vi "Measurement Logic.vi"() -> ()   [LabVIEW 2024, in "Broadband Generation.lvlib"]
uses:
  Broadband Generation.lvlib
  Measurement Results.ctl
  <vilib>/addons/_NISVFA/_Generation/Signal Generation/SV Signal/sv_System Timing Model.ctl
  <vilib>/addons/_NISVFA/_Generation/Signal Generation/SV Signal/SV Signal.lvclass
  <vilib>/addons/_NISVFA/_Generation/Signal Generation/SV Sinusoid/SV Sinusoid.lvclass
  <resource>/objmgr/daqmx.rc
  <vilib>/DAQmx/configure/timing.llb/DAQmx Timing (Sample Clock).vi
  <vilib>/addons/_NISVFA/_Generation/Signal Generation/SV Noise/Configure White Noise.vi
  <vilib>/addons/_NISVFA/_Generation/Signal Generation/SV Noise/SV Noise.lvclass
  <vilib>/DAQmx/create/channels.llb/DAQmx Create Channel (AO-Voltage-Basic).vi
  <vilib>/DAQmx/write.llb/DAQmx Write (Analog 1D Wfm NChan NSamp).vi
  <vilib>/addons/_NISVFA/_Generation/Signal Generation/SV Noise/Configure Pink Noise.vi
  <vilib>/addons/_NISVFA/_Generation/Signal Generation/SV Noise/Configure Periodic Random Noise.vi
  <vilib>/addons/_NISVFA/_Generation/Signal Generation/SV MLS/Configure Maximum Length Sequence.vi
  <vilib>/addons/_NISVFA/_Generation/Signal Generation/SV MLS/SV MLS.lvclass
  <vilib>/Plug-In SDKs/Measurements/Measure Call Context/Measure Call Context.lvclass
  Measurement Configuration.ctl
panel:
  out "measurement results":T1
  in  "measurement configuration":T2={"sample rate"=51200.0, "physical channels"=["Dev1/ao0"], "ranges"=[3.16], "terminal cfgs"=[-1], "type"=[0], "levels"=[0.5]} {"type" items=["White Noise", "Pink Noise", "Periodic Random Noise", "Maximum Length Sequence"]}
  out "measure call context out":refnum<class "Measure Call Context.lvclass">
  in  "measure call context in":refnum<class "Measure Call Context.lvclass">
  out "error out":errorcluster
  in  "error in":errorcluster
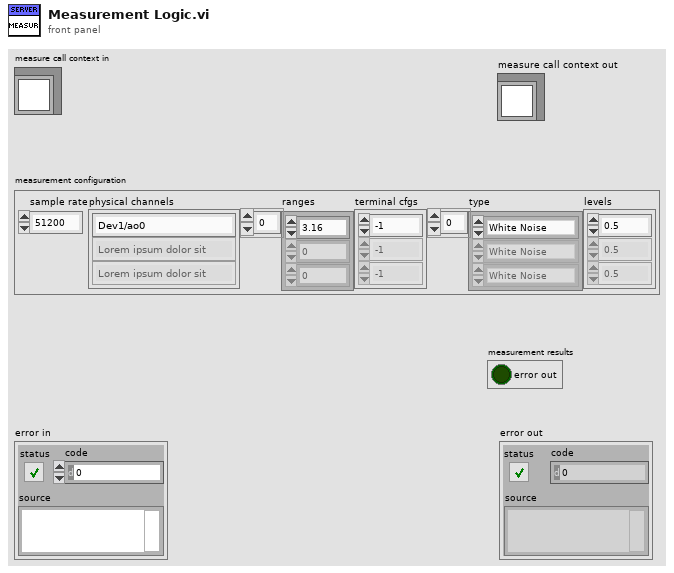
[diagram p1: front panel]
types:
  T1 = typedef "Broadband Generation.lvlib/Measurement Results.ctl" = cluster{"error out":bool}
  T2 = typedef "Broadband Generation.lvlib/Measurement Configuration.ctl" = cluster{"sample rate":dbl, "physical channels":string[], "ranges":dbl[], "terminal cfgs":i32[], "type":i32[], "levels":dbl[]}
  T3 = cluster{"profile":enum16{"Linear", "Half cosine"}, "durations [s]":cluster{"ramp-up":dbl, "transition":dbl, "ramp-down":dbl}}
  T4 = typedef "SV Signal.lvclass/sv_System Timing Model.ctl" = i64
  T5 = typedef "Event Messenger-bool.lvlib/))Channel.ctl" = refnum<queue>
  T6 = typedef "Tag-bool.lvlib/))Channel.ctl" = refnum<queue>
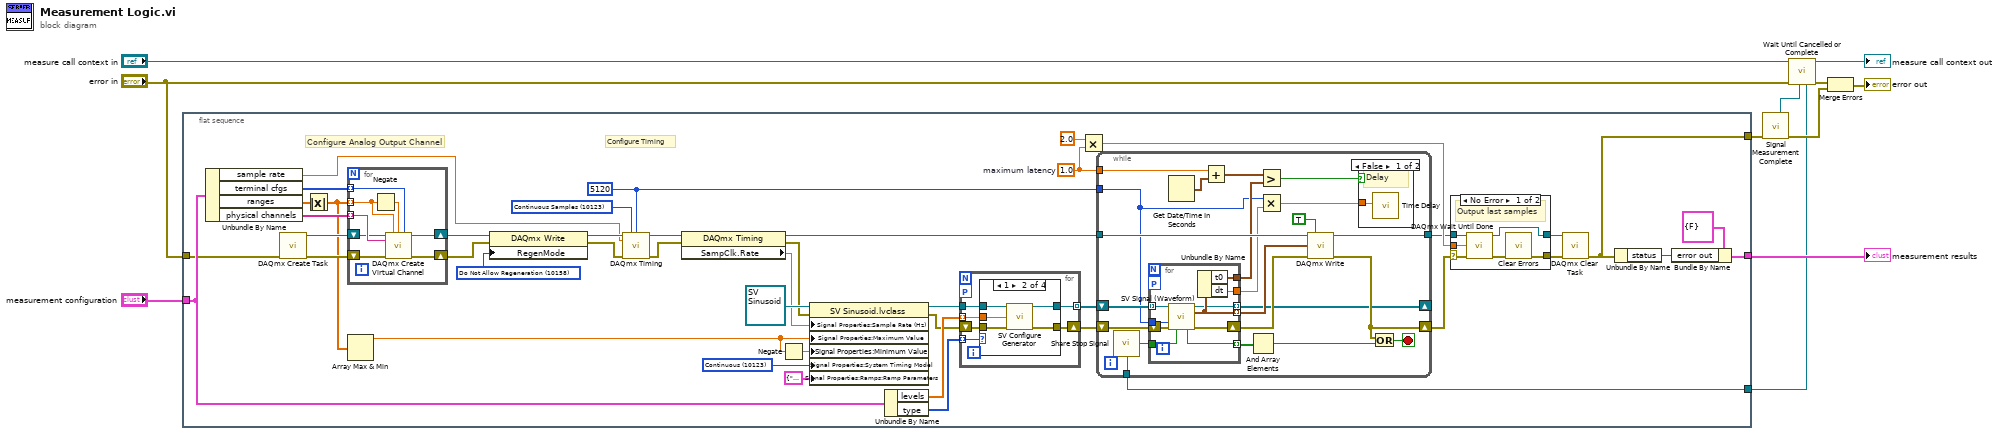
[diagram p0: block diagram]
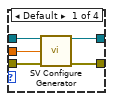
[diagram p4: hidden frame]
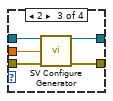
[diagram p5: hidden frame]
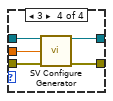
[diagram p6: hidden frame]
diagram:
  n1 = flat-sequence {
    tunnel: "measurement configuration" -> [w53]
    tunnel: [w55] -> w5
    tunnel: "error in" -> [w23]
    tunnel: [w20] -> w3
    tunnel: w4 -> [w24]
    frame #0 {
      w35 = 10158 items=["Allow Regeneration"=10097, "Do Not Allow Regeneration"=10158] ("RegenMode")
      w18 = 5120 ("samples per channel")
      w43 = 10123 items=["Finite Samples"=10178, "Continuous Samples"=10123, "Hardware Timed Single Point"=12522] ("sample mode")
      w28 = 1.0  # maximum latency
      w54 = T4 10123 items=["Finite"=10178, "-"=-1, "Continuous"=10123, "-"=-2, "Settled"=110123, "Averaged"=210123, "Discrete Sweep"=310123, "Continuous Sweep"=410123] ("System Timing Model")
      # "Configure Timing"
      # "Configure Analog Output Channel"
      n2 = Unbundle By Name(w53) -> ("sample rate"=w22:dbl, "terminal cfgs"=w36:i32[], "ranges"=w15:dbl[], "physical channels"=w37:string[])
      n3 = call <vilib>:"DAQmx Create Task.vi"("error in"=w23) -> ("task out"=w34:refnum<k21>, "error out"=w33:errorcluster)  [unwired: 13 in]
      n4 = Absolute Value(x=w15) -> (abs(x)=w14:dbl[])
      n5 = for {
        tunnel: w37 -> [w101] mode=indexing
        tunnel: w14 -> [w100] mode=indexing
        tunnel: w36 -> [w99] mode=indexing
        shift-right: [w103] -> w41
        shift-left: w34 -> [w98]
        shift-right: [w102] -> w39
        shift-left: w33 -> [w97]
        n6 = Negate(x=w100) -> (-x=w104:dbl)
        n7 = call-poly <vilib>:"DAQmx Create Virtual Channel.vi"("task in"=w98, "maximum value"=w100, "minimum value"=w104, "output terminal configuration"=w99, "physical channels"=w101, "error in"=w97) -> ("task out"=w103:refnum<k21>, "error out"=w102:errorcluster)  [unwired: 8 in]
      }
      n8 = Array Max & Min(array=w14) -> (max value=w12:dbl)  [unwired: 3 out]
      n9 = property class="DAQmx Write"(reference=w41, error in=w39, "RegenMode"=w35) -> (reference out=w40:refnum<k21>, error out=w38:errorcluster)
      n10 = call-poly <vilib>:"DAQmx Timing.vi"("task/channels in"=w40, "sample mode"=w43, "samples per channel"=w18, "rate"=w22, "error in"=w38) -> ("task out"=w44:refnum<k21>, "error out"=w42:errorcluster)  [unwired: 9 in]
      n11 = property class="DAQmx Timing"(reference=w44, error in=w42) -> (reference out=w27:refnum<k21>, error out=w31:errorcluster, "SampClk.Rate"=w32:dbl)
      n12 = Negate(x=w12) -> (-x=w13:dbl)
      n13 = property class="SV Sinusoid.lvclass"(reference=refnum<class "SV Sinusoid.lvclass"> refnum ("signal configuration"), error in=w31, "Signal Properties:Sample Rate (Hz)"=w32, "Signal Properties:Maximum Value"=w12, "Signal Properties:Minimum Value"=w13, "Signal Properties:System Timing Model"=w54, "Signal Properties:Ramps:Ramp Parameters"=T3 {"profile"=enum."Half cosine", "durations [s]"={"ramp-up"=0.01, "transition"=0.0, "ramp-down"=0.01}} ("Ramp Parameters:All Elements")) -> (reference out=w51:refnum<class "SV Sinusoid.lvclass">, error out=w48:errorcluster)
      n14 = Unbundle By Name(w53) -> ("levels"=w50:dbl[], "type"=w49:i32[])
      n15 = for {
        tunnel: w51 -> [w110]
        tunnel: w50 -> [w105] mode=indexing
        tunnel: w49 -> [w106] mode=indexing
        tunnel: [w109] -> w47 mode=indexing
        workers-P: _ -> [_]
        shift-right: [w108] -> w46
        shift-left: w48 -> [w107]
        n16 = case shown="1" w106 {
          tunnel: w110 -> [w115 w120 w125 w130]
          tunnel: [w114 w119 w124 w129] -> w109
          tunnel: [w113 w118 w123 w128] -> w108
          tunnel: w107 -> [w112 w117 w122 w127]
          tunnel: w105 -> [w111 w116 w121 w126]
          frame Default {
            n17 = call-poly <vilib>:"SV Configure Generator.vi"("template configuration"=w115, "level"=w111, "error in (no error)"=w112) -> ("signal configuration"=w114:refnum<class "SV Noise.lvclass">, "error out"=w113:errorcluster)  [unwired: 11 in]
          }
          frame 1 {
            n18 = call-poly <vilib>:"SV Configure Generator.vi"("template configuration"=w120, "level"=w116, "error in"=w117) -> ("signal configuration"=w119:refnum<class "SV Noise.lvclass">, "error out"=w118:errorcluster)  [unwired: 11 in]
          }
          frame 2 {
            n19 = call-poly <vilib>:"SV Configure Generator.vi"("template configuration"=w125, "level"=w121, "error in (no error)"=w122) -> ("signal configuration"=w124:refnum<class "SV Noise.lvclass">, "error out"=w123:errorcluster)  [unwired: 11 in]
          }
          frame 3 {
            n20 = call-poly <vilib>:"SV Configure Generator.vi"("template configuration"=w130, "amplitude"=w126, "error in (no error)"=w127) -> ("signal configuration"=w129:refnum<class "SV MLS.lvclass">, "error out"=w128:errorcluster)  [unwired: 11 in]
          }
        }
      }
      n21 = Multiply(x=2.0 ("value"), y=w28) -> (x*y=w29:dbl)
      n22 = while {
        tunnel: w28 -> [w59]
        tunnel: w27 -> [w73]
        shift-right: [w65] -> w25
        shift-left: w46 -> [w76]
        tunnel: [w70] -> w26
        tunnel: w24 -> [w69]
        shift-right: [w63] -> _
        shift-left: w47 -> [w77]
        tunnel: w18 -> [w56]
        stop <- w66 stop-if-true
        n23 = call <vilib>:"Share Stop Signal.vi"("channel"=w69) -> ("stop"=w68:bool)  [unwired: 1 in]
        n24 = for {
          tunnel: [w86] -> w74 mode=indexing
          workers-P: _ -> [_]
          tunnel: w77 -> [w88] mode=indexing
          tunnel: [w85] -> w57
          shift-right: [w84] -> w71
          shift-left: w76 -> [w87]
          tunnel: w68 -> [w83]
          tunnel: [w82] -> w67 mode=indexing
          tunnel: [w81] -> w63 mode=indexing
          tunnel: w56 -> [w80]
          tunnel: [w79] -> w62
          n25 = call-dynamic "SV Signal (Waveform).vi"("signal configuration"=w88, "samples"=w80, "error in (no error)"=w87, "stop"=w83) -> ("signal configuration"=w81:refnum<class "SV Signal.lvclass">, "output waveform"=w86:waveform(dbl), "done"=w82:bool, "error out"=w84:errorcluster)  [unwired: 6 in, 2 out]
          n26 = Unbundle By Name(w86) -> ("t0"=w85:timestamp, "dt"=w79:dbl)
        }
        n27 = Get Date/Time In Seconds() -> (seconds since 1Jan1904=w60:timestamp)
        n28 = Add(x=w59, y=w60) -> (x+y=w58:timestamp)
        n29 = And Array Elements(Boolean array=w67) -> (logical AND=w64:bool)
        n30 = Greater?(x=w58, y=w57) -> (0:w75:bool)
        n31 = Multiply(x=w56, y=w62) -> (x*y=w61:dbl)
        n32 = call-poly <vilib>:"DAQmx Write.vi"("task/channels in"=w73, "auto start"=TRUE, "data"=w74, "error in"=w71) -> ("task out"=w70:refnum<k21>, "error out"=w65:errorcluster)  [unwired: 9 in, 1 out]
        n33 = case shown="False" w75 {
          tunnel: w61 -> [w78 _]
          frame False {
            # "Delay"
            n34 = call "Time Delay"("Delay Time (s)"=w78) -> ()  [unwired: 10 in, 1 out]
          }
          frame True {
            # "Continue"
          }
        }
        n35 = Or(x=w65, y=w64) -> (x .or. y?=w66:bool)
      }
      n36 = case shown="No Error" w25 {
        selector: w25 -> [w93 w96]
        tunnel: w26 -> [w94 w95]
        tunnel: w29 -> [w92 _]
        tunnel: [w91 w96] -> w21
        tunnel: [w89 w95] -> w19
        frame No Error {
          # "Output last samples"
          n37 = call <vilib>:"DAQmx Wait Until Done.vi"("task/channels in"=w94, "timeout (sec)"=w92, "error in"=w93) -> ("task out"=w89:refnum<k21>, "error out"=w90:errorcluster)  [unwired: 11 in]
          n38 = call <vilib>:"Clear Errors.vi"("error in (no error)"=w90) -> ("error out"=w91:errorcluster)  [unwired: 5 in, 1 out]
        }
        frame Error {
          # "Error"
        }
      }
      n39 = call <vilib>:"DAQmx Clear Task.vi"("task in"=w19, "error in"=w21) -> ("error out"=w20:errorcluster)  [unwired: 13 in]
      n40 = Unbundle By Name(w20) -> ("status"=w45:bool)
      n41 = Bundle By Name(cluster=T1 {"error out"=FALSE} ("Measurement Results"), "error out"=w45) -> (w55:T1)
    }
  }
  n42 = call "Signal Measurement Complete.vi"("error in (no error)"=w3) -> ("error out"=w8:errorcluster, "done channel"=w9:T5)  [unwired: 9 in]
  n43 = call "Wait Until Cancelled or Complete.vi"("done channel"=w9, "error in (no error)"="error in", "measure call context in"="measure call context in") -> ("error out"=w7:errorcluster, "measure call context out"=→"measure call context out":refnum<class "Measure Call Context.lvclass">, "channel"=w4:T6)  [unwired: 6 in]
  n44 = Merge Errors(w7, w8) -> (→"error out":errorcluster)
  "measurement results" <- w5
